vi "Find Selected Channel.vi"(8 "error in (no error)":errorcluster, 11 "WaveformProcessor in":refnum<class "WaveformProcessor.lvclass">) -> (0 "error out":errorcluster, 3 "WaveformProcessor out":refnum<class "WaveformProcessor.lvclass">)   [LabVIEW 2019, in "Variant Parser.lvlib" / "WaveformProcessor.lvclass"]
uses:
  Library/WaveformProcessor.lvclass
  Library/WaveformProcessor.lvclass/WaveformProcessor.ctl
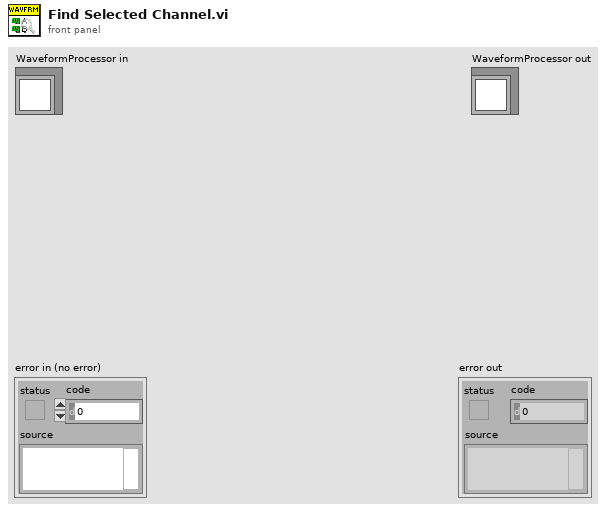
[diagram p1: front panel]
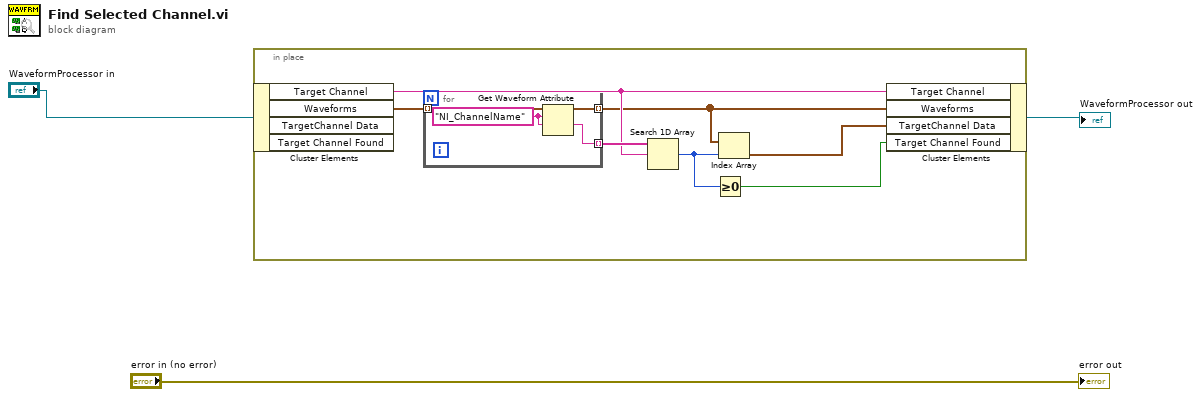
[diagram p0: block diagram]
diagram:
  n1 = in-place {
    n2 = in-place-cluster #1("WaveformProcessor in") -> ("Target Channel"=w8:string, "Waveforms"=w10:waveform(dbl)[])  [unwired: 2 out]
    n3 = for {
      tunnel: w10 -> [w13] mode=indexing
      tunnel: [w12] -> w7 mode=indexing
      tunnel: [w11] -> w9 mode=indexing
      w14 = "NI_ChannelName" ("name")
      n4 = Get Waveform Attribute(5:w14, 6:w14, 7:w13) -> (1:w11:string, 3:w12:waveform(dbl))  [unwired: 1 in, 2 out]
    }
    n5 = Search 1D Array(1D array=w9, element=w8) -> (index of element=w6:i32)  [unwired: 1 in]
    n6 = Greater Or Equal To 0?(x=w6) -> (x >= 0?=w4:bool)
    n7 = Index Array(array=w7, index=w6) -> (element=w5:waveform(dbl))
    n8 = in-place-cluster #1("Target Channel"=w8, "Waveforms"=w7, "TargetChannel Data"=w5, "Target Channel Found"=w4) -> (→"WaveformProcessor out":refnum<class "WaveformProcessor.lvclass">)
  }
  "error out" <- "error in (no error)"
